vi "Imaq_detect_circle_for_TV_coord_1511_1526.vi"(0 "Image":T2, 1 "ROI":T3, 2 "ROI1":T1, 5 "error in (no error)":errorcluster) -> (14 "Image Out":T2(plugin-control), 15 "New Reference":T4 {"Axis Reference" items=["Direct", "Indirect"]; "Angle (deg)" format="%.2f"; "Origin"."Y" format="%.2f"; "Origin"."X" format="%.2f"}, 19 "error out":errorcluster)   [LabVIEW 2019, in "Algorithm.lvclass"]
uses:
  FrameworkOverrides/Algorithm.lvclass
  <vilib>/vision/NI_Vision_Development_Module.lvlib
  <vilib>/vision/Pattern Matching.llb/IMAQ Match Range Setting.ctl
  <vilib>/vision/Shape Detection.llb/ShapeDetectionMatchOptions.ctl
  <vilib>/vision/Pattern Matching.llb/IMAQ Curve Parameters.ctl
  <vilib>/vision/Image Controls.llb/IMAQ Image.ctl
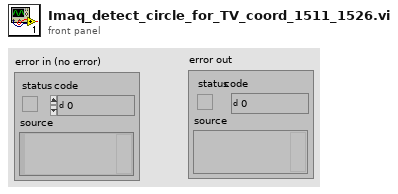
[diagram p1: front panel]
types:
  T1 = cluster{"ROI":cluster{"Left":i32, "Top":i32, "Right":i32, "Bottom":i32, "Rotation":dbl}, "EdgeOptions":cluster{"EdgePolarity":i32, "KernelSize":i32, "Width":i32, "MinimumEdgeStrength":i32, "InterpolationType":i32, "DataProcessingMethod":i32}, "LineOptions":cluster{"NumberofLines":i32, "Type":i32, "MinScore":i32, "MaxScore":i32, "Orientation":i32, "AngleRange":i32, "AngleTolerance":i32, "StepSize":i32, "MinSNR":i32, "MinPoints":i32, "HoughIterations":i32}, "Process":i32, "StepSize":i32, "SearchDirection":i32, "CircleEdgeOptions":cluster{"SearchDirection":i32, "EdgeOptions":cluster{"EdgePolarity":i32, "KernelSize":i32, "Width":i32, "MinimumEdgeStrength":i32, "InterpolationType":i32, "DataProcessingMethod":i32}}, "CircleFitOptions":cluster{"Process":i32, "StepSize":i32, "MAxPixelRadius":i32}, "CircleSearchDirection":i32, "CurveParameters":cluster{"ExtractionMode":i32, "EdgeThreshold":i32, "EdgeFilterSize":i32, "MinLength":i32, "RowSearchStepSize":i32, "ColSearchStepSize":i32, "MaxEndpointGap":i32, "Closed":bool, "Subpixel":bool}, "MinimumMatchScore":i32, "CircleDescriptor":cluster{"MinRadius":i32, "MaxRadius":i32}, "EllipseDescriptor":cluster{"MinMajorRadius":i32, "MaxMajorRadius":i32, "MinMinorRadius":i32, "MaxMinorRadius":i32}, "ParallelLines":cluster{"First":i32, "Second":i32, "Third":i32}}
  T2 = typedef "IMAQ Image.ctl" = refnum<image>
  T3 = cluster{"Global Rectangle":i32[], "Contours":cluster{"Contour Type":u32, "ROI Type":u32, "Points":i32[]}[]}
  T4 = cluster{"Origin":cluster{"X":sgl, "Y":sgl}, "Angle (deg)":sgl, "Axis Reference":u32}
  T5 = typedef "ShapeDetectionMatchOptions.ctl" = cluster{"Rotation":bool, "Scale":bool, "Occlusion":bool, "Range Settings":T6[]}
  T6 = typedef "IMAQ Match Range Setting.ctl" = cluster{"Match Constraints":u32, "Min":dbl, "Max":dbl}
  T7 = cluster{"Point 1":cluster{"X":sgl, "Y":sgl}, "Point 2":cluster{"X":sgl, "Y":sgl}}
  T8 = typedef "IMAQ Curve Parameters.ctl" = cluster{"Extraction Mode":u32, "Edge Threshold":i32, "Edge Filter Size":u32, "Min Length":i32, "Row Search Step Size":i32, "Col Search Step Size":i32, "Max Endpoint Gap":i32, "Closed":bool, "Subpixel":bool}
  T9 = cluster{"EdgePolarity":i32, "KernelSize":i32, "Width":i32, "MinimumEdgeStrength":i32, "InterpolationType":i32, "DataProcessingMethod":i32}
  T10 = cluster{"NumberofLines":i32, "Type":i32, "MinScore":i32, "MaxScore":i32, "Orientation":i32, "AngleRange":i32, "AngleTolerance":i32, "StepSize":i32, "MinSNR":i32, "MinPoints":i32, "HoughIterations":i32}
  T11 = cluster{"ExtractionMode":i32, "EdgeThreshold":i32, "EdgeFilterSize":i32, "MinLength":i32, "RowSearchStepSize":i32, "ColSearchStepSize":i32, "MaxEndpointGap":i32, "Closed":bool, "Subpixel":bool}
  T12 = cluster{"Point1 (Pixels)":cluster{"X":sgl, "Y":sgl}, "Point2 (Pixels)":cluster{"X":sgl, "Y":sgl}, "Point1 (Real-World)":cluster{"X":sgl, "Y":sgl}, "Point2 (Real-World)":cluster{"X":sgl, "Y":sgl}, "Angle (Pixel)":dbl, "Angle (Real-World)":dbl, "Score":dbl, "Straightness":dbl, "Average SNR (db)":dbl, "Calibration Valid":bool}[]
  T13 = typedef "Search Line.ctl" = cluster{"Start Point":cluster{"X":sgl, "Y":sgl}, "End Point":cluster{"X":sgl, "Y":sgl}, "Edge Info":T14[], "Edge Map":dbl[], "Calibration Valid":bool}
  T14 = typedef "Edge New.ctl" = cluster{"Location (Pixel)":cluster{"X":sgl, "Y":sgl}, "Location (Real-World)":cluster{"X":sgl, "Y":sgl}, "Distance (Pixel)":dbl, "Distance (Real-World)":dbl, "Strength":dbl, "Noise":dbl, "Rising?":bool}
  T15 = cluster{"Point1 (Pixels)":cluster{"X":sgl, "Y":sgl}, "Point2 (Pixels)":cluster{"X":sgl, "Y":sgl}, "Point1 (Real-World)":cluster{"X":sgl, "Y":sgl}, "Point2 (Real-World)":cluster{"X":sgl, "Y":sgl}, "Angle (Pixel)":dbl, "Angle (Real-World)":dbl, "Score":dbl, "Straightness":dbl, "Average SNR (db)":dbl, "Calibration Valid":bool}
  T16 = cluster{"Position":cluster{"X":sgl, "Y":sgl}, "Radius":dbl, "Score":dbl}[]
  T17 = cluster{"Position":cluster{"X":sgl, "Y":sgl}, "Radius":dbl, "Score":dbl}
  T18 = cluster{"Point 2":cluster{"X":sgl, "Y":sgl}, "Point 1":cluster{"X":sgl, "Y":sgl}, "Point1 (Pixels)":cluster{"X":sgl, "Y":sgl}}
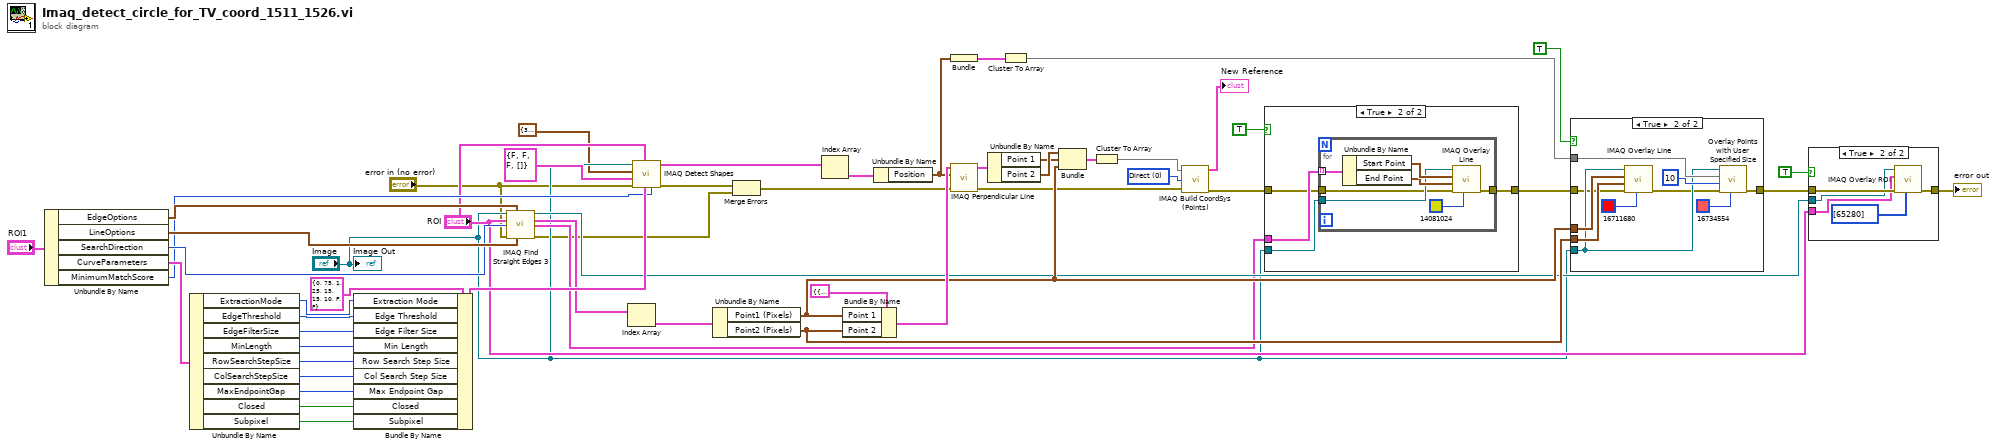
[diagram p0: block diagram]
diagram:
  w31 = u32 0 items=["Direct", "Indirect"] ("Axis Reference")
  n1 = Unbundle By Name("ROI1") -> ("EdgeOptions"=w53:T9, "LineOptions"=w52:T10, "SearchDirection"=w51:i32, "CurveParameters"=w49:T11, "MinimumMatchScore"=w40:i32)
  n2 = Unbundle By Name(w49) -> ("ExtractionMode"=w42:i32, "EdgeThreshold"=w43:i32, "EdgeFilterSize"=w44:i32, "MinLength"=w45:i32, "RowSearchStepSize"=w46:i32, "ColSearchStepSize"=w47:i32, "MaxEndpointGap"=w48:i32, "Closed"=w10:bool, "Subpixel"=w9:bool)
  n3 = Bundle By Name(cluster=T8 {"Extraction Mode"=0, "Edge Threshold"=75, "Edge Filter Size"=1, "Min Length"=25, "Row Search Step Size"=15, "Col Search Step Size"=15, "Max Endpoint Gap"=10, "Closed"=FALSE, "Subpixel"=FALSE} ("Curve Parameters"), "Extraction Mode"=w42, "Edge Threshold"=w43, "Edge Filter Size"=w44, "Min Length"=w45, "Row Search Step Size"=w46, "Col Search Step Size"=w47, "Max Endpoint Gap"=w48, "Closed"=w10, "Subpixel"=w9) -> (w41:T8)
  n4 = call "IMAQ Find Straight Edges 3"("Image"="Image", "Edge Options"=w53, "ROI Descriptor"="ROI", "Search Direction"=w51, "error in (no error)"="error in (no error)", "Line Options"=w52) -> ("Image (duplicate)"=w20:T2, "Straight Edges"=w37:T12, "Search Lines Information"=w18:T13[], "error out"=w7:errorcluster)  [unwired: 5 in, 1 out]
  n5 = Index Array(array=w37) -> (element=w35:T15)  [unwired: 1 in]
  n6 = call-poly "IMAQ Detect Shapes"("Minimum match score"=w40, "Curve Parameters"=w41, "ROI Descriptor"="ROI", "error in (no error)"="error in (no error)", "Match Options"=T5 {"Rotation"=FALSE, "Scale"=FALSE, "Occlusion"=FALSE, "Range Settings"=[]}, "Circle Descriptor"=cluster{"Min Radius":dbl, "Max Radius":dbl} {"Min Radius"=3.0, "Max Radius"=500.0}, "Image"="Image") -> ("error out"=w36:errorcluster, "Circles"=w28:T16)  [unwired: 2 in, 1 out]
  n7 = Unbundle By Name(w35) -> ("Point1 (Pixels)"=w23:cluster{"X":sgl, "Y":sgl}, "Point2 (Pixels)"=w30:cluster{"X":sgl, "Y":sgl})
  n8 = Merge Errors(w36, w7) -> (w4:errorcluster)
  n9 = Index Array(array=w28) -> (element=w38:T17)  [unwired: 1 in]
  n10 = Bundle By Name(cluster=T7 {"Point 1"={"X"=0.0, "Y"=0.0}, "Point 2"={"X"=0.0, "Y"=0.0}} ("Line"), "Point 1"=w23, "Point 2"=w30) -> (w33:T7)
  n11 = Unbundle By Name(w38) -> ("Position"=w27:cluster{"X":sgl, "Y":sgl})
  n12 = Bundle("Position"=w27) -> (w26:cluster{"Position":cluster{"X":sgl, "Y":sgl}})  [unwired: 1 in]
  n13 = call "IMAQ Perpendicular Line"("error in (no error)"=w4, "Point"=w27, "Line"=w33) -> ("error out"=w3:errorcluster, "Perpendicular Line"=w32:T7)  [unwired: 6 in, 1 out]
  n14 = Unbundle By Name(w32) -> ("Point 1"=w24:cluster{"X":sgl, "Y":sgl}, "Point 2"=w25:cluster{"X":sgl, "Y":sgl})
  n15 = Cluster To Array(cluster=w26) -> (array=w16:cluster{"X":sgl, "Y":sgl}[])
  n16 = Bundle("Point 2"=w25, "Point 1"=w24, "Point1 (Pixels)"=w23) -> (w22:T18)  [unwired: 1 in]
  n17 = Cluster To Array(cluster=w22) -> (array=w21:cluster{"X":sgl, "Y":sgl}[])
  n18 = call "IMAQ Build CoordSys (Points)"("Reference Points"=w21, "Axis Reference"=w31, "error in (no error)"=w3) -> ("Coordinate System"=→"New Reference":T4, "error out"=w6:errorcluster)  [unwired: 2 in]
  n19 = case shown="True" TRUE {
    tunnel: w18 -> [_ w58]
    tunnel: "Image" -> [_ w57]
    tunnel: w6 -> [w54 w56]
    tunnel: [w54 w55] -> w5
    frame False {
    }
    frame True {
      n20 = for {
        tunnel: w58 -> [w65] mode=indexing
        tunnel: w57 -> [w61]
        tunnel: w56 -> [w60]
        tunnel: [w59] -> w55
        n21 = Unbundle By Name(w65) -> ("Start Point"=w64:cluster{"X":sgl, "Y":sgl}, "End Point"=w63:cluster{"X":sgl, "Y":sgl})
        n22 = call "IMAQ Overlay Line"("Color"=u32 14081024, "error in (no error)"=w60, "End Point"=w63, "Start Point"=w64, "Image"=w61) -> ("error out"=w59:errorcluster)  [unwired: 5 in, 1 out]
      }
    }
  }
  n23 = case shown="True" TRUE {
    tunnel: w30 -> [_ w75]
    tunnel: w23 -> [_ w74]
    tunnel: "Image" -> [_ w70]
    tunnel: w16 -> [_ w71]
    tunnel: w5 -> [w66 w69]
    tunnel: [w66 w67] -> w2
    frame False {
    }
    frame True {
      n24 = call "IMAQ Overlay Line"("Color"=u32 16711680, "error in (no error)"=w69, "End Point"=w75, "Start Point"=w74, "Image"=w70) -> ("error out"=w68:errorcluster)  [unwired: 5 in, 1 out]
      n25 = call "Overlay Points with User Specified Size.vi"("Color"=u32 16734554, "error in"=w68, "Point Diameter (5)"=u32 10, "Points"=w71, "Image In"=w70) -> ("error out"=w67:errorcluster)  [unwired: 5 in, 1 out]
    }
  }
  n26 = case shown="True" TRUE {
    tunnel: w2 -> [w77 w82]
    tunnel: [w77 w81] -> w1
    tunnel: w20 -> [_ w80]
    tunnel: "ROI" -> [_ w79]
    frame False {
    }
    frame True {
      n27 = call "IMAQ Overlay ROI"("Colors (Green)"=u32[] [65280], "error in (no error)"=w82, "ROI Descriptor"=w79, "Image"=w80) -> ("error out"=w81:errorcluster)  [unwired: 6 in, 1 out]
    }
  }
  "error out" <- w1
  "Image Out" <- "Image"
